vi "GamepiecePose.vi"(2 "tx(deg)":dbl, 3 "ty(deg)":dbl, 4 "piece":string) -> (0 "Gamepiece_Y":dbl, 1 "Gamepiece_X":dbl)   [LabVIEW 2020]
uses:
  GlobalPoseAndTargeting.vi
panel:
  out "Vision Valid?":bool
  out "range_center(in)":dbl
  out "range_front(in)":dbl
  out "x distance front(in)":dbl
  out "y distance front (in)":dbl
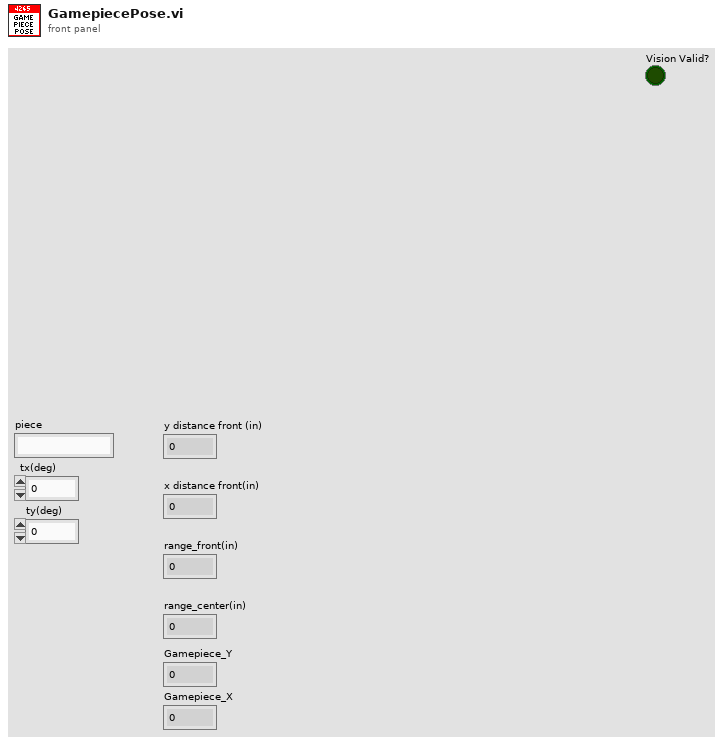
[diagram p1: front panel]
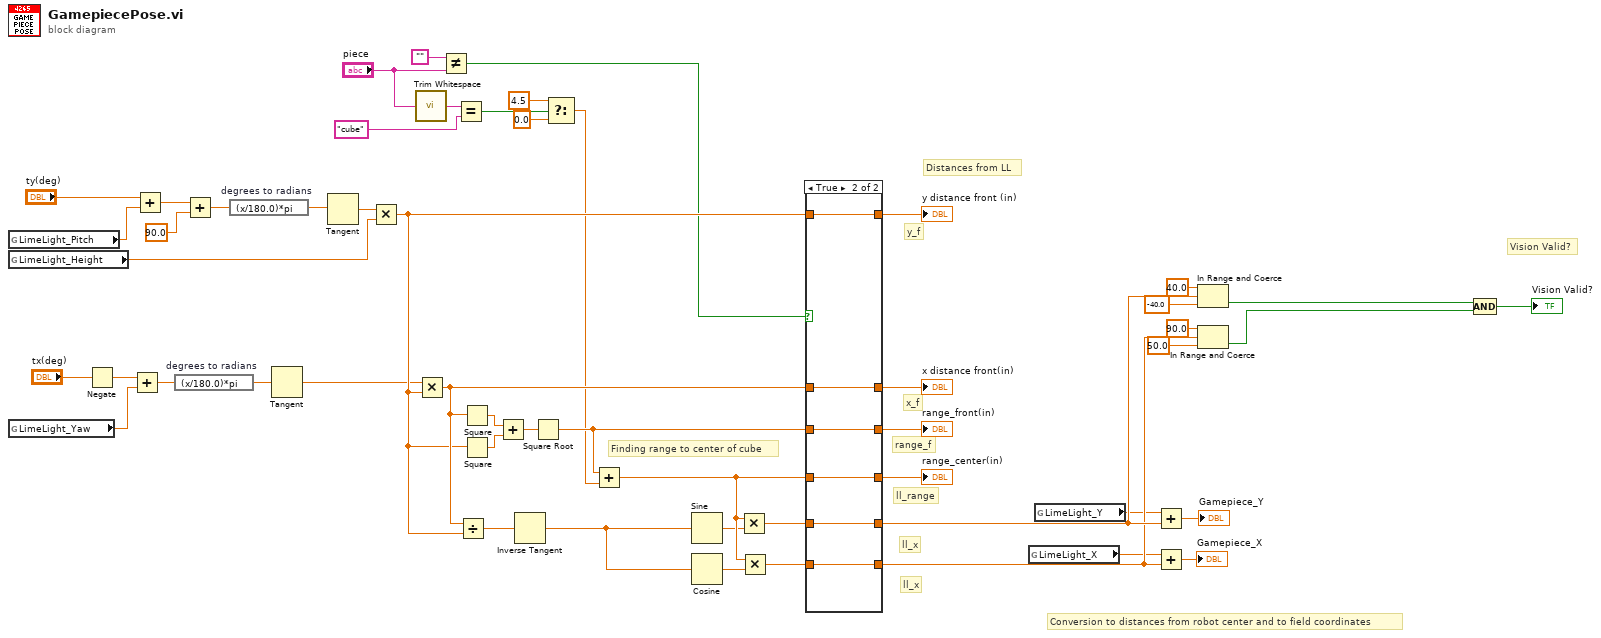
[diagram p0: block diagram]
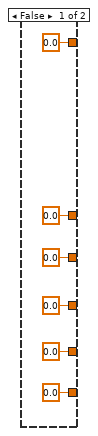
[diagram p2: hidden frame]
diagram:
  # "Vision Valid?"
  # "ll_x"
  # "ll_x"
  # "ll_range"
  # "range_f"
  # "x_f"
  # "y_f"
  # "Conversion to distances from robot center and to field coordinates"
  # "Distances from LL"
  # "Finding range to center of cube"
  n1 = global read "GlobalPoseAndTargeting.vi" "LimeLight_Pitch"() -> (w17:dbl)
  n2 = global read "GlobalPoseAndTargeting.vi" "LimeLight_Height"() -> (w15:dbl)
  n3 = global read "GlobalPoseAndTargeting.vi" "LimeLight_Yaw"() -> (w16:dbl)
  n4 = Negate(x="tx(deg)") -> (-x=w1:dbl)
  n5 = Add(x=w1, y=w16) -> (x+y=w31:dbl)
  n6 = Add(x="ty(deg)", y=w17) -> (x+y=w28:dbl)
  n7 = expression code="(x/180.0)*pi" "degrees to radians"(w31) -> (w32:dbl)
  n8 = Add(x=w28, y=90.0) -> (x+y=w29:dbl)
  n9 = expression code="(x/180.0)*pi" "degrees to radians"(w29) -> (w27:dbl)
  n10 = Tangent(1:w32) -> (0:w33:dbl)
  n11 = Tangent(1:w27) -> (0:w26:dbl)
  n12 = Multiply(x=w26, y=w15) -> (x*y=w45:dbl)
  n13 = call <vilib>:"Trim Whitespace.vi"("string"="piece") -> ("trimmed string"=w20:string)  [unwired: 1 in]
  n14 = Multiply(x=w33, y=w45) -> (x*y=w47:dbl)
  n15 = Not Equal?(x="", y="piece") -> (x != y?=w23:bool)
  n16 = Equal?(x=w20, y="cube") -> (x = y?=w18:bool)
  n17 = Divide(x=w47, y=w45) -> (x/y=w37:dbl)
  n18 = Square(x=w47) -> (x^2=w34:dbl)
  n19 = Square(x=w45) -> (x^2=w35:dbl)
  n20 = Add(x=w34, y=w35) -> (x+y=w36:dbl)
  n21 = Inverse Tangent(1:w37) -> (0:w39:dbl)
  n22 = Square Root(x=w36) -> (sqrt(x)=w49:dbl)
  n23 = Select(t=4.5 ("y"), s=w18, f=0.0) -> (s? t:f=w42:dbl)
  n24 = Add(x=w49, y=w42) -> (x+y=w50:dbl)
  n25 = Sine(x=w39) -> (sin(x)=w38:dbl)
  n26 = Cosine(x=w39) -> (cos(x)=w40:dbl)
  n27 = Multiply(x=w50, y=w38) -> (x*y=w52:dbl)
  n28 = Multiply(x=w50, y=w40) -> (x*y=w53:dbl)
  n29 = case shown="True" w23 {
    tunnel: [0.0 w65] -> w44
    tunnel: w45 -> [_ w65]
    tunnel: [0.0 w64] -> w46
    tunnel: w47 -> [_ w64]
    tunnel: [0.0 w63] -> w48
    tunnel: w49 -> [_ w63]
    tunnel: w50 -> [_ w62]
    tunnel: [0.0 w62] -> w51
    tunnel: w52 -> [_ w61]
    tunnel: [0.0 w61] -> w12
    tunnel: w53 -> [_ w60]
    tunnel: [0.0 w60] -> w11
    frame False {
    }
    frame True {
    }
  }
  "y distance front (in)" <- w44
  "x distance front(in)" <- w46
  "range_front(in)" <- w48
  "range_center(in)" <- w51
  n30 = global read "GlobalPoseAndTargeting.vi" "LimeLight_X"() -> (w2:dbl)
  n31 = global read "GlobalPoseAndTargeting.vi" "LimeLight_Y"() -> (w3:dbl)
  n32 = Add(x=w3, y=w12) -> (x+y=→"Gamepiece_Y":dbl)
  n33 = Add(x=w2, y=w11) -> (x+y=→"Gamepiece_X":dbl)
  n34 = In Range and Coerce(upper limit=40.0, x=w12, lower limit=-40.0) -> (In Range?=w9:bool)  [unwired: 1 out]
  n35 = In Range and Coerce(upper limit=90.0, x=w11, lower limit=50.0) -> (In Range?=w8:bool)  [unwired: 1 out]
  n36 = Compound Arithmetic op=AND(w9, w8) -> (→"Vision Valid?":bool)
